vi "Reference_Inst_Info_2_string.vi"(1 "Ref Instrument type":T1=enum."LDA", 2 "Calib filename":path, 3 "Port":string, 4 "Device":string, 5 "Ch No":i16, 6 "Reference Name":string="Instrument to calibrate") -> (0 "Setup String":string)   [LabVIEW 2021]
uses:
  Controls/Ref_Inst_type.ctl
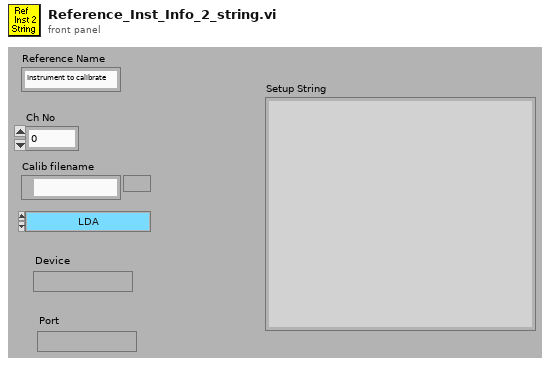
[diagram p1: front panel]
types:
  T1 = typedef "Ref_Inst_type.ctl" = enum16{"Propellor anemometer", "Pressure Transducer", "Raw voltage", "Pitot-static tube", "Generic Linear", "Generic Polynomial", "Thermocouple", "LDA", "Enter Value", "ADAM Channel"}
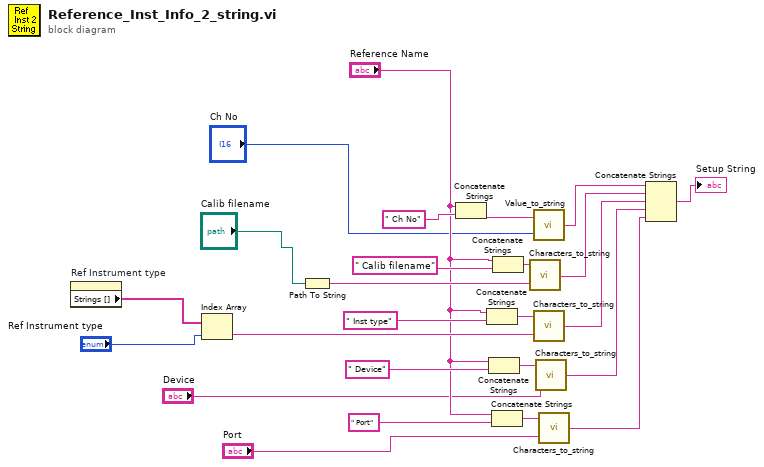
[diagram p0: block diagram]
diagram:
  n1 = property on="Ref Instrument type" class="Enum (strict)"() -> ("Strings []"=w20:string[])  [unwired: 2 in, 2 out]
  n2 = Index Array(array=w20, index="Ref Instrument type") -> (element=w19:string)
  n3 = Path To String(path="Calib filename") -> (string=w23:string)
  n4 = Concatenate Strings("Reference Name", " Ch No") -> (w24:string)
  n5 = Concatenate Strings("Reference Name", " Inst type") -> (w17:string)
  n6 = Concatenate Strings("Reference Name", " Device") -> (w12:string)
  n7 = Concatenate Strings("Reference Name", " Port") -> (w9:string)
  n8 = Concatenate Strings("Reference Name", " Calib filename") -> (w22:string)
  n9 = call "Characters_to_string.vi"("Characters to write"=w23, "Label for characters"=w22) -> ("Output string"=w15:string)  [unwired: 1 in]
  n10 = call "Value_to_string.vi"("Value"="Ch No", "Label for value"=w24) -> ("Output string"=w16:string)  [unwired: 1 in]
  n11 = call "Characters_to_string.vi"("Characters to write"=w19, "Label for characters"=w17) -> ("Output string"=w14:string)  [unwired: 1 in]
  n12 = call "Characters_to_string.vi"("Characters to write"="Device", "Label for characters"=w12) -> ("Output string"=w7:string)  [unwired: 1 in]
  n13 = call "Characters_to_string.vi"("Characters to write"="Port", "Label for characters"=w9) -> ("Output string"=w6:string)  [unwired: 1 in]
  n14 = Concatenate Strings(w16, w15, w14, w7, w6) -> (→"Setup String":string)
